vi "HOST.vi"() -> ()   [LabVIEW 2018]
uses:
  <vilib>/userdefined/High Color/nirio_resource_hc.ctl
  <instrlib>/niDCPower/nidcpower.llb/niDCPower Measurement Type.ctl
  <vilib>/FPGAPlugInAG/PXI-7953R/niLvFpga_Open_PXI-7953R.vi
  <vilib>/rvi/interface/common/dynamic/niFpgaDynamicAddResources.vi
  <vilib>/FPGAPlugInAG/Dynamic/niLvFpga_Reset_Dynamic.vi
  <vilib>/FPGAPlugInAG/Dynamic/niLvFpga_Run_Dynamic.vi
  <vilib>/Utility/error.llb/Error Cluster From Error Code.vi
  <vilib>/rvi/errors/niLvFpgaAdjustHostInterfaceError.vi
  <vilib>/FPGAPlugInAG/Dynamic/niLvFpga_Close_Dynamic.vi
  <vilib>/rvi/interface/nirviOpenFPGA/nirviOpenFPGA.xnode
  FPGA Bitfiles/MT9V024IA7XTM_FPGATarget_Target_SM0JNh2yPhg.lvbitx
  <vilib>/rvi/interface/nirviMethod/nirviMethod.xnode
  <vilib>/rvi/interface/nirviReadWriteControl/nirviReadWriteControl.xnode
  <vilib>/rvi/interface/nirviCloseFPGA/nirviCloseFPGA.xnode
  <vilib>/rvi/interface/Simulation/niFpgaSimulationCallBeginRW.vi
  <vilib>/FPGAPlugInAG/Dynamic/niLvFpga_ReadFifo_Dynamic.vi
  <vilib>/rvi/errors/niLvFpgaMergeErrorWithErrorCode.vi
  NiFpgaLv.dll
  <vilib>/Analysis/NI_AALBase.lvlib
panel:
  in  "Tab Control":enum32{"Основной", "Служебный"}(tab)
  out "Номер образца":string="0"
  in  "SEL 2":path=path "C:/LabView_PRJ/MT9V024IA7XTM/SEL"
  in  "resource name":T1="PXI1Slot6"
  in  "VAA_PIX":refnum<k15>="PXI1Slot3" caption="instrument handle"
  in  "VDD_LVDS":refnum<k15>="PXI1Slot2" caption="instrument handle"
  in  "Стоп":bool
  in  "Питание":bool
  out "VDD Chart":dbl(graph)=-7.930775234089577 caption="Waveform Chart 5"
  out "VAA Chart":dbl(graph)=0.06968054713639742
  out "LVDS Chart":dbl(graph)=0.00048817553524479985
  out "VAA_cur, A":dbl caption="measurement" format="%_6g"
  in  "VAA_curlim, A":dbl=0.1 caption="current limit" format="%_6p"
  in  "VAA, V":dbl=3.3 caption="voltage level" format="%_6p"
  in  "LVDS, V":dbl=3.3 caption="voltage level" format="%_6p"
  out "LVDS_cur, A":dbl caption="measurement" format="%_6g"
  out "VDD_cur, A":dbl caption="measurement" format="%_6g"
  in  "LVDS_curlim, A":dbl=0.1 caption="current limit" format="%_6p"
  in  "VDD_curlim, A":dbl=0.1 caption="current limit" format="%_6p"
  in  "VDD, V":dbl=3.3 caption="voltage level" format="%_6p"
  out "PIX Chart":dbl(graph)=-0.009814653457617957
  out "PIX_cur, A":dbl caption="measurement" format="%_6g"
  in  "PIX_curlim, A":dbl=0.1 caption="current limit" format="%_6p"
  in  "PIX, V":dbl=3.3 caption="voltage level" format="%_6p"
  in  "ON/OFF":bool
  in  "STANDBY":bool
  in  "nRESET_BAR":bool
  in  "VDD_selcur":dbl=0.075 caption="current limit" format="%_6p"
  in  "LVDS_selcur":dbl=0.075 caption="current limit" format="%_6p"
  in  "VAA_selcur":dbl=0.075 caption="current limit" format="%_6p"
  in  "PIX_selcur":dbl=0.075 caption="current limit" format="%_6p"
  out "VDD 2":bool
  out "LVDS 2":bool
  out "VAA 2":bool
  out "PIX 2":bool
  out "VDD":u32
  out "LVDS":u32
  out "VAA":u32
  out "PIX":u32
  in  "Период, мс":u32=100
  in  "SIM_SEL":bool
  out "SEL":bool
  out "REG_WR":bool
  in  "Получить кадр":bool
  in  "Непрерывно":bool=TRUE
  in  "SEL_T, мс":u32=100
  in  "Прошивка":bool
  in  "SAVE":bool
  in  "ПРИМЕЧАНИЕ":string
  in  "Светлый (T)\nТемный (F)":bool
  in  "Запись(T)/Чтение(F)":bool
  out "Image":T2(plugin-control)
  out "READ":u16=16 format="%x"
  in  "Регистр":u8=7 format="%x"
  in  "Данные":u16=920 format="%x"
  in  "Запись":u16=184 format="%x"
  out "Записали адресов":u32=360960
  out "世男":bool
  in  "Frames":path=path "C:/LabView_PRJ/MT9V024IA7XTM/FRAMES"
  out "СКО, ед.":u16=13
  out "СЗ, ед":u16=891
  in  "Со стороны":bool
  in  "Анализ":path=path "C:/Users/agest/Downloads/MT9V024IA7XTM/MT9V024IA7XTM/FRAMES/Первый кадр.PNG"
  in  "Write":bool[](array[boolean])=[FALSE, FALSE, FALSE, FALSE, FALSE, FALSE, FALSE, FALSE, TRUE, FALSE, FALSE, TRUE, TRUE, TRUE, FALSE, TRUE, FALSE, FALSE, TRUE, FALSE, FALSE, TRUE, FALSE, FALSE, FALSE, FALSE, FALSE, FALSE, FALSE, FALSE, TRUE, TRUE, TRUE, FALSE, TRUE]
  out "Array":bool[](array[boolean])=[TRUE, TRUE, TRUE, TRUE, TRUE, TRUE, TRUE, TRUE, FALSE, FALSE, FALSE, FALSE, FALSE, FALSE, FALSE, FALSE, FALSE, FALSE, TRUE, TRUE, FALSE, TRUE, FALSE, FALSE, FALSE, FALSE, FALSE, FALSE, FALSE, FALSE, TRUE, TRUE, TRUE, FALSE, TRUE, FALSE, FALSE, FALSE, FALSE, FALSE, FALSE, FALSE, FALSE]
  out "Read":bool[](array[boolean])=[FALSE, FALSE, FALSE, FALSE, TRUE, FALSE, FALSE, FALSE, TRUE, FALSE, FALSE, FALSE, FALSE, FALSE, FALSE, FALSE, FALSE]
  out "array w/ subset deleted":bool[](array[boolean])=[FALSE, FALSE, FALSE, FALSE, TRUE, FALSE, FALSE, FALSE, FALSE, FALSE, FALSE, FALSE, FALSE, FALSE, FALSE, FALSE]
  in  "Адресмассив":u8[](array[numeric])=[7, 175, 32, 112, 13, 15] format="%x"
  in  "Данныемассив":u16[](array[numeric])=[920, 0, 453, 1, 784, 257] format="%x"
  out "Data":u16[][](array[numeric])
  # "7 - 398\nAF - 0\n20 - 1C5\n70 - 1\nD - 310\nB - 10 (1 мс)\nB - 627 (100 мс)"
  # "D0"
  # "D7"
  # "\"0\""
  # "D8"
  # "D15"
  # "\"0\""
  # "R0"
  # "R7"
  # "\"0\""
  # "А0"
  # "\"В8\" - запись"
  # "А7"
  # "А0"
  # "St"
  # "\"0\""
  # "R0"
  # "R7"
  # "\"0\""
  # "А0"
  # "\"В8\" - запись"
  # "А7"
  # "А7"
  # "\"В9\" - чтение"
  # "0"
  # "35"
  # "Режим \"Запись\""
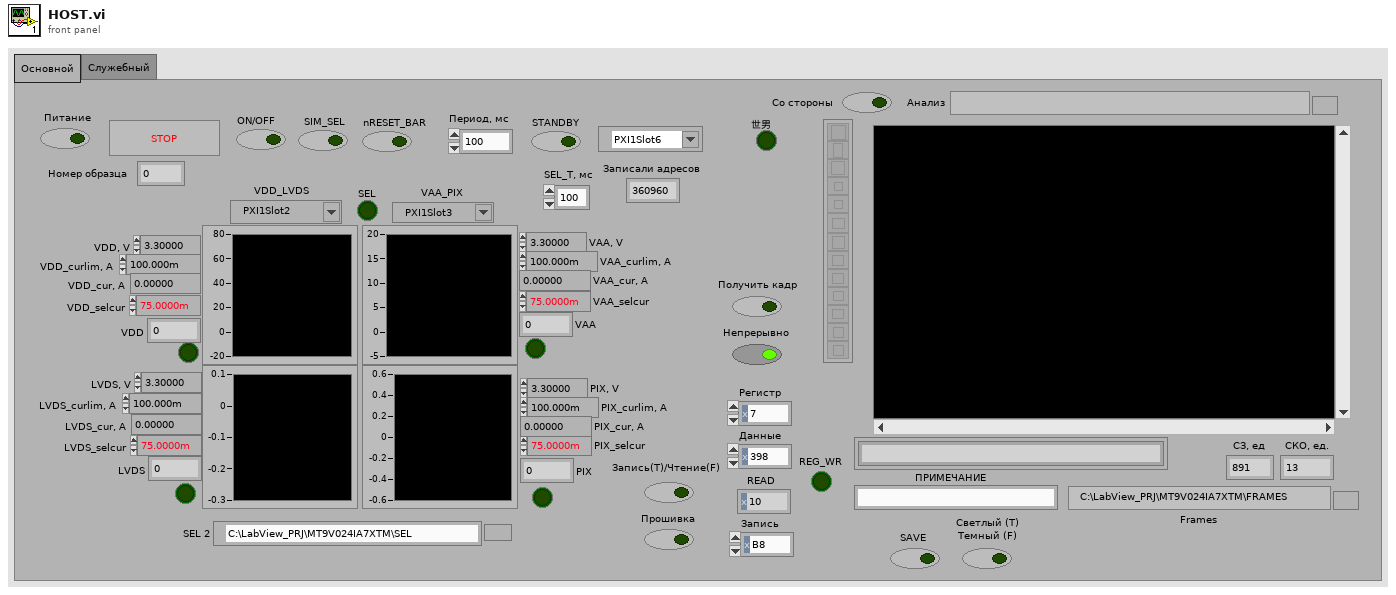
[diagram p1: front panel]
types:
  T1 = typedef "nirio_resource_hc.ctl" = tag
  T2 = typedef "IMAQ Image.ctl" = refnum<image>
  T3 = typedef "Image Type" = u32
  T4 = enum16{"open", "replace", "create", "open or create", "replace or create", "replace or create with confirmation"}
  T5 = typedef "niDCPower Measurement Type.ctl" = i32
  T6 = cluster{"Global Rectangle":i32[], "Contours":cluster{"Contour Type":u32, "ROI Type":u32, "Points":i32[]}[]}
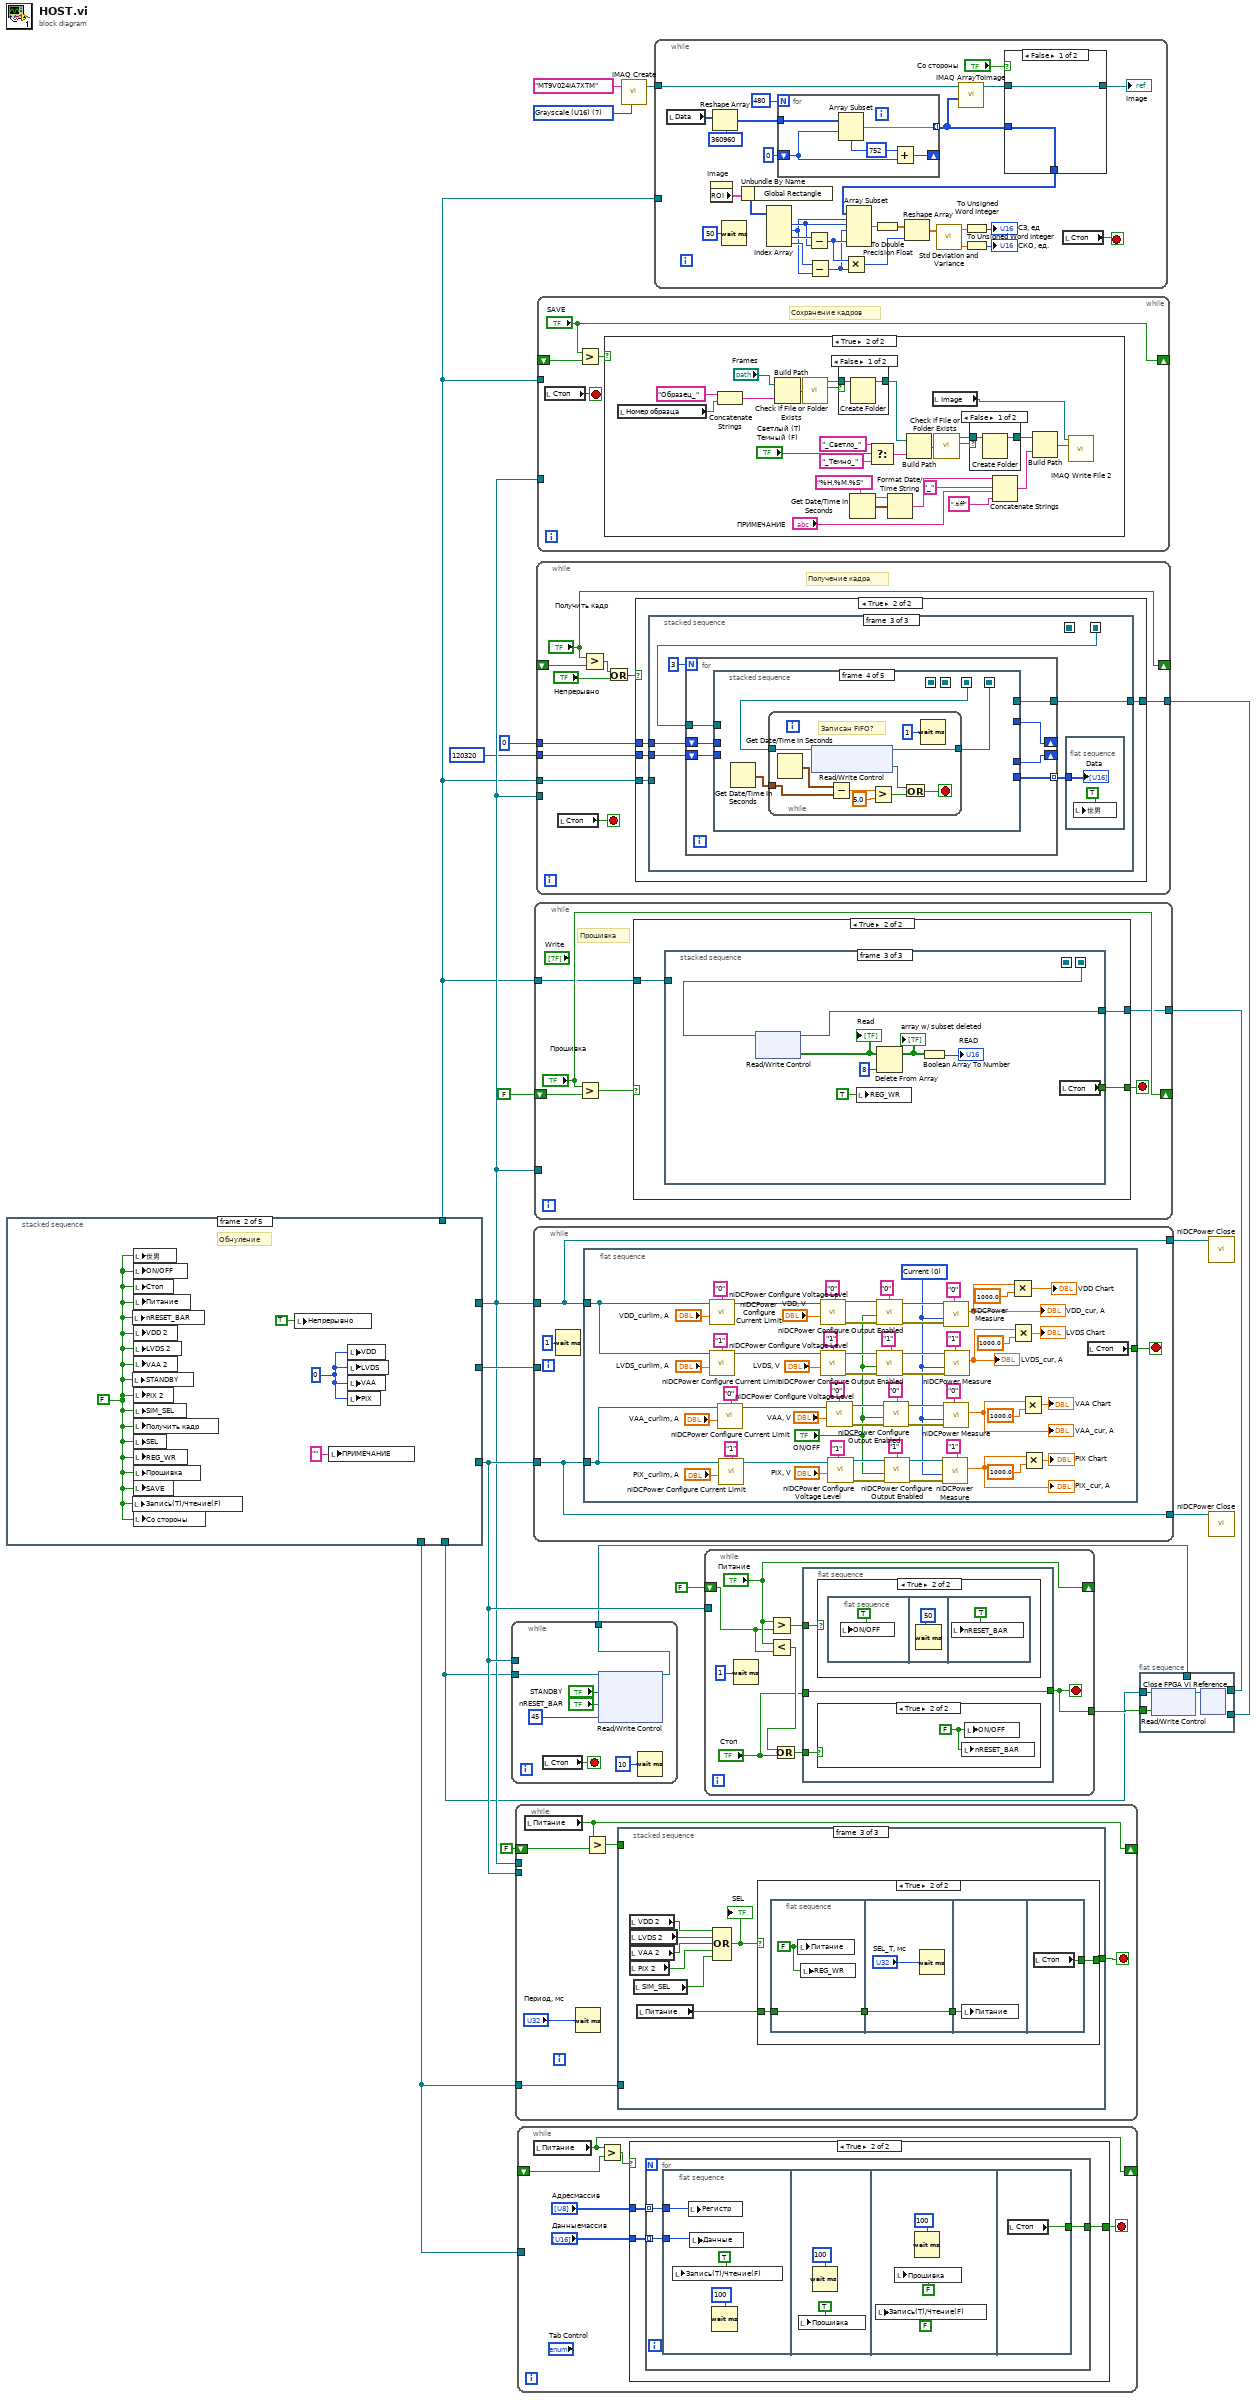
[diagram p0: block diagram]
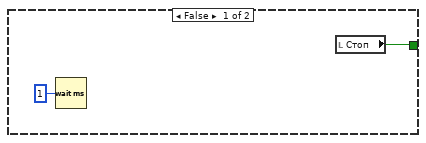
[diagram p2: hidden frame]
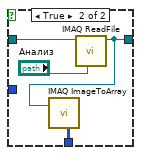
[diagram p3: hidden frame]
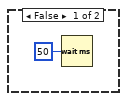
[diagram p4: hidden frame]
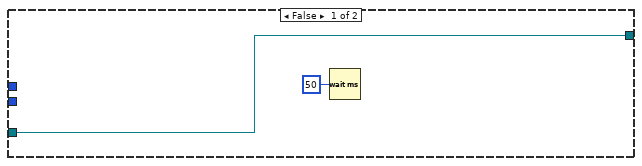
[diagram p7: hidden frame]
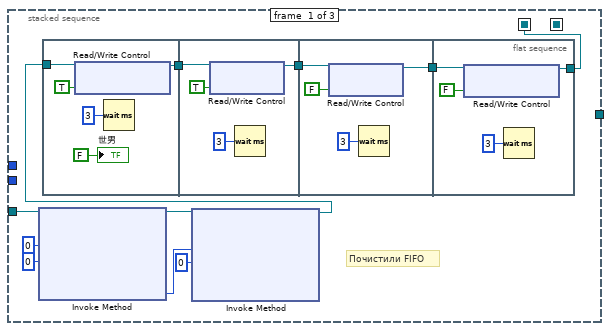
[diagram p8: hidden frame]
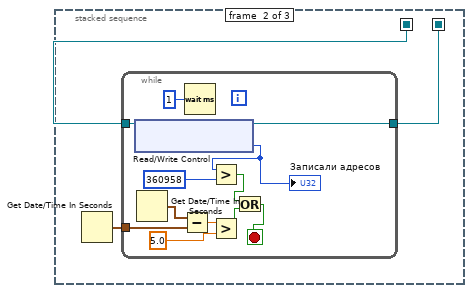
[diagram p9: hidden frame]
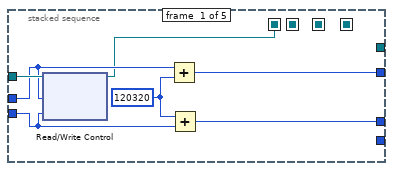
[diagram p10: hidden frame]
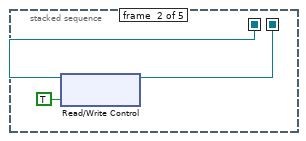
[diagram p11: hidden frame]
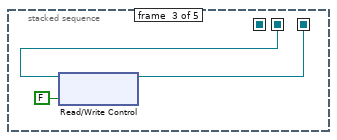
[diagram p12: hidden frame]
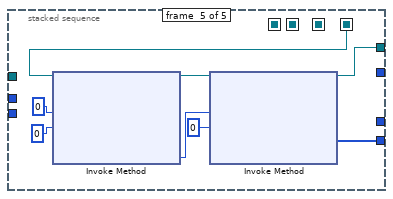
[diagram p13: hidden frame]
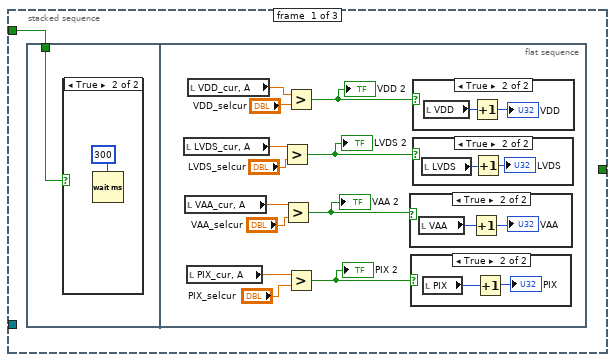
[diagram p14: hidden frame]
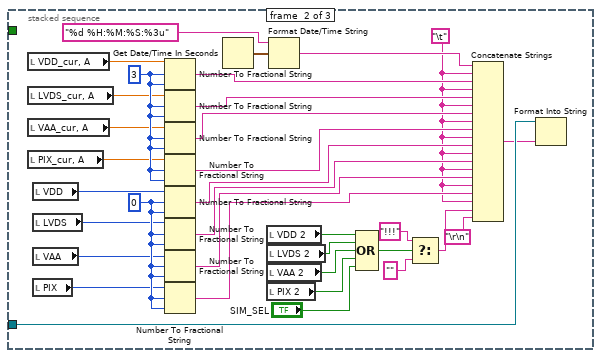
[diagram p20: hidden frame]
diagram:
  w8 = T3 7 items=["Grayscale (U8)", "Grayscale (I16)", "Grayscale (SGL)", "Complex (CSG)", "RGB (U32)", "HSL (U32)", "RGB (U64)", "Grayscale (U16)"] ("Image Type")
  n1 = stacked-sequence {
    tunnel: [_ _ w26 _ _] -> w3
    tunnel: [_ _ _ w62 _] -> w13
    tunnel: [_ _ _ _ w69] -> w12
    tunnel: [_ _ _ _ w68] -> w16
    tunnel: [_ _ _ w62 _] -> w4
    tunnel: [_ _ _ w62 _] -> w2
    frame #0 {
      # "Begin"
      n2 = call "Begin.vi"() -> ("Номер образца 2"=→"Номер образца":string)  [unwired: 11 in]
    }
    frame #1 {
      w25 = u32 0
      w22 = FALSE
      # "Обнуление"
      n3 = local write "nRESET_BAR"(w22) -> ()
      n4 = local write "STANDBY"(w22) -> ()
      n5 = local write "Запись(T)/Чтение(F)"(w22) -> ()
      n6 = local write "世男"(w22) -> ()
      n7 = local write "ON/OFF"(w22) -> ()
      n8 = local write "Стоп"(w22) -> ()
      n9 = local write "Питание"(w22) -> ()
      n10 = local write "VDD 2"(w22) -> ()
      n11 = local write "LVDS 2"(w22) -> ()
      n12 = local write "VAA 2"(w22) -> ()
      n13 = local write "PIX 2"(w22) -> ()
      n14 = local write "SIM_SEL"(w22) -> ()
      n15 = local write "Получить кадр"(w22) -> ()
      n16 = local write "SEL"(w22) -> ()
      n17 = local write "REG_WR"(w22) -> ()
      n18 = local write "Прошивка"(w22) -> ()
      n19 = local write "SAVE"(w22) -> ()
      n20 = local write "Со стороны"(w22) -> ()
      n21 = local write "Непрерывно"(TRUE ("Непрерывно")) -> ()
      n22 = local write "ПРИМЕЧАНИЕ"("" ("ПРИМЕЧАНИЕ")) -> ()
      n23 = local write "VDD"(w25) -> ()
      n24 = local write "LVDS"(w25) -> ()
      n25 = local write "VAA"(w25) -> ()
      n26 = local write "PIX"(w25) -> ()
    }
    frame #2 {
      w29 = "\t"
      # "Инициализаци первой строки лога по токам"
      n27 = local read "Номер образца"() -> (w35:string)
      n28 = Build Path(base path="SEL 2", name or relative path=w35) -> (appended path=w33:path)
      n29 = Get Date/Time In Seconds() -> (seconds since 1Jan1904=w40:timestamp)
      n30 = call <vilib>:"Check if File or Folder Exists.vi"("path"=w33) -> ("file or folder exists?"=w32:bool, "dup path"=w31:path)  [unwired: 8 in, 1 out]
      n31 = Format Date/Time String(time format string (%c)="%d %H.%M.%S", seconds (now)=w40) -> (date/time string=w43:string)  [unwired: 1 in]
      n32 = case shown="False" w32 {
        tunnel: w31 -> [w60 w61]
        tunnel: [w59 w61] -> w47
        frame False {
          n33 = Create Folder(path (use dialog)=w60) -> (created path=w59:path)  [unwired: 2 in, 2 out]
        }
        frame True {
        }
      }
      n34 = Concatenate Strings(w43, ".xls" ("string")) -> (w45:string)
      n35 = Build Path(base path=w47, name or relative path=w45) -> (appended path=w42:path)
      n36 = Open/Create/Replace File(file path (use dialog)=w42, operation (0:open)=T4."open or create", access (0:read/write)=enum16{"read/write", "read-only", "write-only"}."read/write") -> (refnum out=w39:refnum<file>)  [unwired: 3 in, 2 out]
      n37 = case shown="True" TRUE {
        tunnel: w39 -> [w55 w58]
        tunnel: [w55 w56] -> w46
        frame False {
        }
        frame True {
          n38 = Set File Position(refnum=w58, from (0:start)=enum16{"start", "end", "current"}."end") -> (refnum out=w56:refnum<file>)  [unwired: 2 in, 1 out]
        }
      }
      n39 = Format Into String(initial string=w46, "Time" ("input 1"), w29, "VDD_cur" ("input 1"), w29, "VDDLVDS_cur" ("input 1"), w29, "VAA_cur" ("input 1"), w29, "VAAPIX_cur" ("input 1"), w29, "VDD_sel" ("input 1"), w29, "VDDLVDS_sel" ("input 1"), w29, "VAA_sel" ("input 1"), w29, "VAAPIX_sel" ("input 1"), "\r\n") -> (resulting string=w26:refnum<file>)  [unwired: 2 in, 1 out]
    }
    frame #3 {
      n40 = xnode "Open FPGA VI Reference"("resource name"="resource name") -> ("FPGA VI Reference Out"=w63:refnum<k20>, "error out"=w65:errorcluster)  [unwired: 1 in]
      n41 = xnode "Invoke Method"("FPGA VI Reference In"=w63, "error in"=w65) -> ("FPGA VI Reference Out"=w66:refnum<k20>, "error out"=w64:errorcluster)
      n42 = xnode "Invoke Method"("FPGA VI Reference In"=w66, "error in"=w64) -> ("FPGA VI Reference Out"=w62:refnum<k20>)  [unwired: 1 in, 1 out]
    }
    frame #4 {
      n43 = call <instrlib>:"niDCPower Initialize.vi"("resource name"="VDD_LVDS") -> ("error out"=w73:errorcluster, "instrument handle out"=w71:refnum<k15>)  [unwired: 3 in, 6 out]
      n44 = call <instrlib>:"niDCPower Initialize.vi"("resource name"="VAA_PIX") -> ("error out"=w72:errorcluster, "instrument handle out"=w70:refnum<k15>)  [unwired: 3 in, 6 out]
      n45 = call <instrlib>:"niDCPower Configure Voltage Level.vi"("error in (no error)"=w73, "voltage level"=0.0, "channel name"="0,1", "instrument handle"=w71) -> ("instrument handle out"=w69:refnum<k15>)  [unwired: 6 in, 1 out]
      n46 = call <instrlib>:"niDCPower Configure Voltage Level.vi"("error in (no error)"=w72, "voltage level"=0.0, "channel name"="0,1", "instrument handle"=w70) -> ("instrument handle out"=w68:refnum<k15>)  [unwired: 6 in, 1 out]
    }
  }
  n47 = while {
    tunnel: w4 -> [w85]
    tunnel: w16 -> [_]
    tunnel: [w80] -> w7
    stop <- w86 stop-if-true
    n48 = local read "Стоп"() -> (w86:bool)
    n49 = xnode "Read/Write Control"("FPGA VI Reference In"=w85, "STANDBY"="STANDBY", "RESET_BAR"="nRESET_BAR", "46"=u8 45) -> ("FPGA VI Reference Out"=w80:refnum<k20>)  [unwired: 1 in, 1 out]
    n50 = Wait (ms)(milliseconds to wait=u32 10) -> ()  [unwired: 1 out]
  }
  n51 = while {
    tunnel: w16 -> [_]
    tunnel: w12 -> [_]
    shift-right: [w91] -> _
    shift-left: FALSE ("Питание") -> [w92]
    tunnel: w3 -> [w87]
    stop <- w89 stop-if-true
    n52 = local read "Питание"() -> (w91:bool)
    n53 = Wait (ms)(milliseconds to wait="Период, мс") -> ()  [unwired: 1 out]
    n54 = Greater?(x=w91, y=w92) -> (0:w90:bool)
    n55 = stacked-sequence {
      tunnel: w90 -> [w93 _ _]
      tunnel: [_ _ w151] -> w89
      tunnel: w87 -> [_ w146 _]
      frame #0 {
        n56 = flat-sequence {
          tunnel: w93 -> [w94]
          frame #0 {
            n57 = case shown="True" w94 {
              frame False {
              }
              frame True {
                n58 = Wait (ms)(milliseconds to wait=u32 300) -> ()  [unwired: 1 out]
              }
            }
          }
          frame #1 {
            n59 = local read "LVDS_cur, A"() -> (w105:dbl)
            n60 = local read "VAA_cur, A"() -> (w103:dbl)
            n61 = local read "PIX_cur, A"() -> (w101:dbl)
            n62 = local read "VDD_cur, A"() -> (w107:dbl)
            n63 = Greater?(x=w105, y="LVDS_selcur") -> (0:w96:bool)
            "LVDS 2" <- w96
            n64 = Greater?(x=w103, y="VAA_selcur") -> (0:w98:bool)
            "VAA 2" <- w98
            n65 = Greater?(x=w107, y="VDD_selcur") -> (0:w97:bool)
            "VDD 2" <- w97
            n66 = Greater?(x=w101, y="PIX_selcur") -> (0:w99:bool)
            "PIX 2" <- w99
            n67 = case shown="True" w98 {
              frame False {
              }
              frame True {
                n68 = local read "VAA"() -> (w113:u32)
                n69 = Increment(x=w113) -> (x+1=→"VAA":u32)
              }
            }
            n70 = case shown="True" w99 {
              frame False {
              }
              frame True {
                n71 = local read "PIX"() -> (w111:u32)
                n72 = Increment(x=w111) -> (x+1=→"PIX":u32)
              }
            }
            n73 = case shown="True" w97 {
              frame False {
              }
              frame True {
                n74 = local read "VDD"() -> (w115:u32)
                n75 = Increment(x=w115) -> (x+1=→"VDD":u32)
              }
            }
            n76 = case shown="True" w96 {
              frame False {
              }
              frame True {
                n77 = local read "LVDS"() -> (w109:u32)
                n78 = Increment(x=w109) -> (x+1=→"LVDS":u32)
              }
            }
          }
        }
      }
      frame #1 {
        w148 = i16 0 ("width (-)")
        w147 = i16 3 ("width (-)")
        w123 = "\t"
        n79 = local read "VDD_cur, A"() -> (w144:dbl)
        n80 = local read "LVDS_cur, A"() -> (w143:dbl)
        n81 = local read "VAA_cur, A"() -> (w142:dbl)
        n82 = local read "PIX_cur, A"() -> (w141:dbl)
        n83 = local read "VDD"() -> (w119:u32)
        n84 = local read "LVDS"() -> (w118:u32)
        n85 = local read "VAA"() -> (w117:u32)
        n86 = local read "PIX"() -> (w116:u32)
        n87 = Number To Fractional String(number=w144, width (-)=w147, precision (6)=w147) -> (F-format string=w131:string)  [unwired: 1 in]
        n88 = Number To Fractional String(number=w143, width (-)=w147, precision (6)=w147) -> (F-format string=w130:string)  [unwired: 1 in]
        n89 = Number To Fractional String(number=w142, width (-)=w147, precision (6)=w147) -> (F-format string=w129:string)  [unwired: 1 in]
        n90 = Number To Fractional String(number=w141, width (-)=w147, precision (6)=w147) -> (F-format string=w128:string)  [unwired: 1 in]
        n91 = Number To Fractional String(number=w119, width (-)=w148, precision (6)=w148) -> (F-format string=w127:string)  [unwired: 1 in]
        n92 = Number To Fractional String(number=w118, width (-)=w148, precision (6)=w148) -> (F-format string=w126:string)  [unwired: 1 in]
        n93 = Number To Fractional String(number=w117, width (-)=w148, precision (6)=w148) -> (F-format string=w125:string)  [unwired: 1 in]
        n94 = Number To Fractional String(number=w116, width (-)=w148, precision (6)=w148) -> (F-format string=w124:string)  [unwired: 1 in]
        n95 = Get Date/Time In Seconds() -> (seconds since 1Jan1904=w145:timestamp)
        n96 = local read "VDD 2"() -> (w140:bool)
        n97 = local read "LVDS 2"() -> (w139:bool)
        n98 = local read "VAA 2"() -> (w138:bool)
        n99 = local read "PIX 2"() -> (w137:bool)
        n100 = Format Date/Time String(time format string (%c)="%d %H:%M:%S:%3u", seconds (now)=w145) -> (date/time string=w132:string)  [unwired: 1 in]
        n101 = Compound Arithmetic op=OR(w140, w139, w138, w137, "SIM_SEL") -> (w133:bool)
        n102 = Select(t="!!!", s=w133, f="") -> (s? t:f=w122:string)
        n103 = Concatenate Strings(w132, w123, w131, w123, w130, w123, w129, w123, w128, w123, w127, w123, w126, w123, w125, w123, w124, w123, w122, "\r\n") -> (w120:string)
        n104 = Format Into String(initial string=w146, w120) -> ()  [unwired: 2 in, 2 out]
      }
      frame #2 {
        n105 = local read "VDD 2"() -> (w157:bool)
        n106 = local read "LVDS 2"() -> (w156:bool)
        n107 = local read "VAA 2"() -> (w155:bool)
        n108 = local read "PIX 2"() -> (w154:bool)
        n109 = local read "SIM_SEL"() -> (w153:bool)
        n110 = local read "Питание"() -> (w150:bool)
        n111 = Compound Arithmetic op=OR(w157, w156, w155, w154, w153) -> (w152:bool)
        "SEL" <- w152
        n112 = case shown="True" w152 {
          tunnel: [w158 w162] -> w151
          tunnel: w150 -> [_ w159]
          frame False {
            n113 = local read "Стоп"() -> (w158:bool)
          }
          frame True {
            n114 = flat-sequence {
              tunnel: [w163] -> w160
              tunnel: w159 -> [w163]
              tunnel: [w165] -> w161
              tunnel: w160 -> [w165]
              tunnel: w161 -> [w167]
              tunnel: [w168] -> w162
              frame #0 {
                w164 = FALSE ("Питание")
                n115 = local write "Питание"(w164) -> ()
                n116 = local write "REG_WR"(w164) -> ()
              }
              frame #1 {
                n117 = Wait (ms)(milliseconds to wait="SEL_T, мс") -> ()  [unwired: 1 out]
              }
              frame #2 {
                n118 = local write "Питание"(w167) -> ()
              }
              frame #3 {
                n119 = local read "Стоп"() -> (w168:bool)
              }
            }
          }
        }
      }
    }
  }
  n120 = while {
    tunnel: w3 -> [_]
    shift-right: [w172] -> _
    shift-left: _ -> [w174]
    stop <- w171 stop-if-true
    n121 = local read "Питание"() -> (w172:bool)
    n122 = Greater?(x=w172, y=w174) -> (0:w173:bool)
    n123 = case shown="True" w173 {
      tunnel: [w175 w179] -> w171
      tunnel: "Адресмассив" -> [_ w178]
      tunnel: "Данныемассив" -> [_ w177]
      frame False {
        n124 = Wait (ms)(milliseconds to wait=u32 1) -> ()  [unwired: 1 out]
        n125 = local read "Стоп"() -> (w175:bool)
      }
      frame True {
        n126 = for {
          tunnel: [w182] -> w179
          tunnel: w178 -> [w181] mode=indexing
          tunnel: w177 -> [w180] mode=indexing
          n127 = flat-sequence {
            tunnel: w181 -> [w184]
            tunnel: w180 -> [w183]
            tunnel: [w192] -> w182
            frame #0 {
              n128 = local write "Запись(T)/Чтение(F)"(TRUE ("Запись(T)/Чтение(F)")) -> ()
              n129 = local write "Регистр"(w184) -> ()
              n130 = local write "Данные"(w183) -> ()
              n131 = Wait (ms)(milliseconds to wait=u32 100) -> ()  [unwired: 1 out]
            }
            frame #1 {
              n132 = local write "Прошивка"(TRUE ("Прошивка")) -> ()
              n133 = Wait (ms)(milliseconds to wait=u32 100) -> ()  [unwired: 1 out]
            }
            frame #2 {
              n134 = local write "Запись(T)/Чтение(F)"(FALSE ("Запись(T)/Чтение(F)")) -> ()
              n135 = local write "Прошивка"(FALSE ("Прошивка")) -> ()
              n136 = Wait (ms)(milliseconds to wait=u32 100) -> ()  [unwired: 1 out]
            }
            frame #3 {
              n137 = local read "Стоп"() -> (w192:bool)
            }
          }
        }
      }
    }
  }
  n138 = while {
    tunnel: w16 -> [w193]
    tunnel: w12 -> [w194]
    tunnel: [w194] -> w18
    tunnel: [w193] -> w19
    tunnel: w13 -> [_]
    stop <- w195 stop-if-true
    n139 = Wait (ms)(milliseconds to wait=u32 1) -> ()  [unwired: 1 out]
    n140 = flat-sequence {
      tunnel: w194 -> [w216]
      tunnel: w193 -> [w202]
      tunnel: [w214] -> w195
      frame #0 {
        w201 = T5 0 items=["Current", "Voltage"] ("measurement type")
        n141 = call <instrlib>:"niDCPower Configure Current Limit.vi"("current limit"="VDD_curlim, A", "channel name"="0", "instrument handle"=w216) -> ("instrument handle out"=w247:refnum<k15>)  [unwired: 7 in, 1 out]
        n142 = call <instrlib>:"niDCPower Configure Current Limit.vi"("current limit"="LVDS_curlim, A", "channel name"="1", "instrument handle"=w216) -> ("instrument handle out"=w248:refnum<k15>)  [unwired: 7 in, 1 out]
        n143 = call <instrlib>:"niDCPower Configure Current Limit.vi"("current limit"="VAA_curlim, A", "channel name"="0", "instrument handle"=w202) -> ("instrument handle out"=w230:refnum<k15>)  [unwired: 7 in, 1 out]
        n144 = call <instrlib>:"niDCPower Configure Current Limit.vi"("current limit"="PIX_curlim, A", "channel name"="1", "instrument handle"=w202) -> ("instrument handle out"=w207:refnum<k15>)  [unwired: 7 in, 1 out]
        n145 = call <instrlib>:"niDCPower Configure Voltage Level.vi"("voltage level"="VDD, V", "channel name"="0", "instrument handle"=w247) -> ("error out"=w240:errorcluster, "instrument handle out"=w243:refnum<k15>)  [unwired: 7 in]
        n146 = call <instrlib>:"niDCPower Configure Voltage Level.vi"("voltage level"="LVDS, V", "channel name"="1", "instrument handle"=w248) -> ("error out"=w241:errorcluster, "instrument handle out"=w242:refnum<k15>)  [unwired: 7 in]
        n147 = call <instrlib>:"niDCPower Configure Voltage Level.vi"("voltage level"="VAA, V", "channel name"="0", "instrument handle"=w230) -> ("error out"=w234:errorcluster, "instrument handle out"=w235:refnum<k15>)  [unwired: 7 in]
        n148 = call <instrlib>:"niDCPower Configure Voltage Level.vi"("voltage level"="PIX, V", "channel name"="1", "instrument handle"=w207) -> ("error out"=w205:errorcluster, "instrument handle out"=w204:refnum<k15>)  [unwired: 7 in]
        n149 = call <instrlib>:"niDCPower Configure Output Enabled.vi"("error in (no error)"=w240, "output enabled"="ON/OFF", "channel name"="0", "instrument handle"=w243) -> ("error out"=w252:errorcluster, "instrument handle out"=w251:refnum<k15>)  [unwired: 6 in]
        n150 = call <instrlib>:"niDCPower Configure Output Enabled.vi"("error in (no error)"=w241, "output enabled"="ON/OFF", "channel name"="1", "instrument handle"=w242) -> ("error out"=w253:errorcluster, "instrument handle out"=w254:refnum<k15>)  [unwired: 6 in]
        n151 = call <instrlib>:"niDCPower Configure Output Enabled.vi"("error in (no error)"=w234, "output enabled"="ON/OFF", "channel name"="0", "instrument handle"=w235) -> ("error out"=w226:errorcluster, "instrument handle out"=w227:refnum<k15>)  [unwired: 6 in]
        n152 = call <instrlib>:"niDCPower Configure Output Enabled.vi"("error in (no error)"=w205, "output enabled"="ON/OFF", "channel name"="1", "instrument handle"=w204) -> ("error out"=w210:errorcluster, "instrument handle out"=w209:refnum<k15>)  [unwired: 6 in]
        n153 = call <instrlib>:"niDCPower Measure.vi"("error in (no error)"=w210, "measurement type"=w201, "channel name"="1", "instrument handle"=w209) -> ("measurement"=w213:dbl)  [unwired: 5 in, 2 out]
        "PIX_cur, A" <- w213
        n154 = call <instrlib>:"niDCPower Measure.vi"("error in (no error)"=w252, "measurement type"=w201, "channel name"="0", "instrument handle"=w251) -> ("measurement"=w219:dbl)  [unwired: 5 in, 2 out]
        "VDD_cur, A" <- w219
        n155 = call <instrlib>:"niDCPower Measure.vi"("error in (no error)"=w226, "measurement type"=w201, "channel name"="0", "instrument handle"=w227) -> ("measurement"=w220:dbl)  [unwired: 5 in, 2 out]
        "VAA_cur, A" <- w220
        n156 = call <instrlib>:"niDCPower Measure.vi"("error in (no error)"=w253, "measurement type"=w201, "channel name"="1", "instrument handle"=w254) -> ("measurement"=w222:dbl)  [unwired: 5 in, 2 out]
        "LVDS_cur, A" <- w222
        n157 = Multiply(x=w219, y=1000.0) -> (x*y=→"VDD Chart":dbl)
        n158 = Multiply(x=w222, y=1000.0) -> (x*y=→"LVDS Chart":dbl)
        n159 = Multiply(x=w220, y=1000.0) -> (x*y=→"VAA Chart":dbl)
        n160 = Multiply(x=w213, y=1000.0) -> (x*y=→"PIX Chart":dbl)
        n161 = local read "Стоп"() -> (w214:bool)
      }
    }
  }
  n162 = while {
    shift-right: ["Прошивка"] -> _
    shift-left: FALSE ("Прошивка") -> [w263]
    tunnel: w12 -> [_]
    tunnel: w2 -> [w260]
    tunnel: [w259] -> w6
    stop <- w261 stop-if-true
    # "Прошивка"
    n163 = Greater?(x="Прошивка", y=w263) -> (0:w258:bool)
    n164 = case shown="True" w258 {
      tunnel: [w265 w269] -> w261
      tunnel: w260 -> [w264 w268]
      tunnel: [w264 w267] -> w259
      frame False {
        n165 = Wait (ms)(milliseconds to wait=u32 1) -> ()  [unwired: 1 out]
        n166 = local read "Стоп"() -> (w265:bool)
      }
      frame True {
        n167 = stacked-sequence {
          seq-local: [w270 _ _] -> [_ w302 _]
          seq-local: [_ w301 _] -> [_ _ w314]
          tunnel: [_ _ w319] -> w269
          tunnel: w268 -> [w288 _ _]
          tunnel: [_ _ w313] -> w267
          frame #0 {
            n168 = Increment(x="Запись") -> (x+1=w272:u16)
            n169 = Multiply(x=u16 256, y=w272) -> (x*y=w281:u16)
            n170 = Number To Boolean Array(number="Запись") -> (Boolean array=w282:bool[])
            n171 = Number To Boolean Array(number="Данные") -> (Boolean array=w279:bool[])
            n172 = Number To Boolean Array(number="Регистр") -> (Boolean array=w283:bool[])
            n173 = Number To Boolean Array(number=w281) -> (Boolean array=w284:bool[])
            n174 = Delete From Array(array=w279, length=8, index=8) -> (deleted portion=w275:bool[], array with subset deleted=w276:bool[])
            n175 = case shown="False" "Запись(T)/Чтение(F)" {
              tunnel: FALSE -> [w291 w297]
              tunnel: w284 -> [w290 _]
              tunnel: w283 -> [w293 w300]
              tunnel: w282 -> [w294 w298]
              tunnel: [w292 w299] -> w280
              tunnel: w276 -> [_ w296]
              tunnel: w275 -> [_ w295]
              frame False {
                n176 = Build Array (concatenate)(w290, w291, w291, w293, w291, w294) -> (w292:bool[])
              }
              frame True {
                n177 = Build Array (concatenate)(w296, w297, w295, w297, w300, w297, w298) -> (w299:bool[])
              }
            }
            "Array" <- w280
            n178 = xnode "Read/Write Control"("FPGA VI Reference In"=w288, "Write"=w280, "Запись(T)/Чтение(F)"="Запись(T)/Чтение(F)") -> ("FPGA VI Reference Out"=w270:refnum<k20>)  [unwired: 1 in, 1 out]
            "REG_WR" <- FALSE ("REG_WR")
          }
          frame #1 {
            # "Цикл записи всех интересующих нас регистров"
            n179 = flat-sequence {
              tunnel: [w306] -> w303
              tunnel: w302 -> [w305]
              tunnel: [w309] -> w304
              tunnel: w303 -> [w309]
              tunnel: w304 -> [w312]
              tunnel: [w310] -> w301
              frame #0 {
                n180 = xnode "Read/Write Control"("FPGA VI Reference In"=w305, "Регистр"=TRUE) -> ("FPGA VI Reference Out"=w306:refnum<k20>)  [unwired: 1 in, 1 out]
              }
              frame #1 {
                n181 = Wait (ms)(milliseconds to wait=u32 1) -> ()  [unwired: 1 out]
              }
              frame #2 {
                n182 = xnode "Read/Write Control"("FPGA VI Reference In"=w312, "Регистр"=FALSE) -> ("FPGA VI Reference Out"=w310:refnum<k20>)  [unwired: 1 in, 1 out]
              }
            }
          }
          frame #2 {
            n183 = xnode "Read/Write Control"("FPGA VI Reference In"=w314) -> ("FPGA VI Reference Out"=w313:refnum<k20>, "Read"=w316:bool[])  [unwired: 1 in, 1 out]
            "Read" <- w316
            n184 = local write "REG_WR"(TRUE ("REG_WR")) -> ()
            n185 = Delete From Array(array=w316, index=8) -> (array with subset deleted=w315:bool[])  [unwired: 1 in, 1 out]
            "array w/ subset deleted" <- w315
            n186 = Boolean Array To Number(Boolean array=w315) -> (number=→"READ":u16)
            n187 = local read "Стоп"() -> (w319:bool)
          }
        }
      }
    }
  }
  n188 = while {
    tunnel: w12 -> [_]
    tunnel: w2 -> [w324]
    shift-right: ["Получить кадр"] -> _
    shift-left: _ -> [w329]
    tunnel: u32 0 -> [w323]
    tunnel: u32 120320 ("163840") -> [w322]
    tunnel: [w321] -> w5
    stop <- w330 stop-if-true
    # "Получение кадра"
    n189 = local read "Стоп"() -> (w330:bool)
    n190 = Greater?(x="Получить кадр", y=w329) -> (0:w326:bool)
    n191 = Or(x=w326, y="Непрерывно") -> (x .or. y?=w325:bool)
    n192 = case shown="True" w325 {
      tunnel: w324 -> [w331 w336]
      tunnel: w323 -> [_ w335]
      tunnel: w322 -> [_ w334]
      tunnel: [w331 w333] -> w321
      frame False {
        n193 = Wait (ms)(milliseconds to wait=u32 50) -> ()  [unwired: 1 out]
      }
      frame True {
        n194 = stacked-sequence {
          seq-local: [w337 _ _] -> [_ w366 _]
          seq-local: [_ w365 _] -> [_ _ w381]
          tunnel: w336 -> [w343 _ _]
          tunnel: w335 -> [_ _ w384]
          tunnel: w334 -> [_ _ w383]
          tunnel: [_ _ w380] -> w333
          frame #0 {
            # "Почистили FIFO"
            n195 = xnode "Invoke Method"("FPGA VI Reference In"=w343, "Number of Elements"=u32 0, "Timeout (ms)"=0) -> ("FPGA VI Reference Out"=w342:refnum<k20>, "Elements Remaining"=w344:u32)  [unwired: 1 in, 2 out]
            n196 = flat-sequence {
              tunnel: w341 -> [w352]
              tunnel: [w349] -> w340
              tunnel: w340 -> [w355]
              tunnel: [w353] -> w339
              tunnel: w339 -> [w359]
              tunnel: [w358] -> w338
              tunnel: w338 -> [w363]
              tunnel: [w361] -> w337
              frame #0 {
                n197 = xnode "Read/Write Control"("FPGA VI Reference In"=w352, "Кадр в память"=TRUE ("EXPOSURE")) -> ("FPGA VI Reference Out"=w349:refnum<k20>)  [unwired: 1 in, 1 out]
                n198 = Wait (ms)(milliseconds to wait=u32 3) -> ()  [unwired: 1 out]
                "世男" <- FALSE
              }
              frame #1 {
                n199 = xnode "Read/Write Control"("FPGA VI Reference In"=w355, "EXPOSURE"=TRUE) -> ("FPGA VI Reference Out"=w353:refnum<k20>)  [unwired: 1 in, 1 out]
                n200 = Wait (ms)(milliseconds to wait=u32 3) -> ()  [unwired: 1 out]
              }
              frame #2 {
                n201 = xnode "Read/Write Control"("FPGA VI Reference In"=w359, "EXPOSURE"=FALSE) -> ("FPGA VI Reference Out"=w358:refnum<k20>)  [unwired: 1 in, 1 out]
                n202 = Wait (ms)(milliseconds to wait=u32 3) -> ()  [unwired: 1 out]
              }
              frame #3 {
                n203 = xnode "Read/Write Control"("FPGA VI Reference In"=w363, "Кадр в память"=FALSE) -> ("FPGA VI Reference Out"=w361:refnum<k20>)  [unwired: 1 in, 1 out]
                n204 = Wait (ms)(milliseconds to wait=u32 3) -> ()  [unwired: 1 out]
              }
            }
            n205 = xnode "Invoke Method"("FPGA VI Reference In"=w342, "Number of Elements"=w344, "Timeout (ms)"=0) -> ("FPGA VI Reference Out"=w341:refnum<k20>)  [unwired: 1 in, 3 out]
          }
          frame #1 {
            n206 = Get Date/Time In Seconds() -> (seconds since 1Jan1904=w367:timestamp)
            n207 = while {
              tunnel: [w378] -> w365
              tunnel: w366 -> [w377]
              tunnel: w367 -> [w374]
              stop <- w369 stop-if-true
              n208 = xnode "Read/Write Control"("FPGA VI Reference In"=w377) -> ("FPGA VI Reference Out"=w378:refnum<k20>, "Записали адресов"=w368:u32)  [unwired: 1 in, 1 out]
              "Записали адресов" <- w368
              n209 = Get Date/Time In Seconds() -> (seconds since 1Jan1904=w375:timestamp)
              n210 = Subtract(x=w375, y=w374) -> (x-y=w373:dbl)
              n211 = Wait (ms)(milliseconds to wait=u32 1) -> ()  [unwired: 1 out]
              n212 = Greater?(x=w368, y=u32 360958) -> (0:w371:bool)
              n213 = Greater?(x=w373, y=5.0) -> (0:w370:bool)
              n214 = Or(x=w371, y=w370) -> (x .or. y?=w369:bool)
            }
          }
          frame #2 {
            n215 = for {
              N: 3 -> [_]
              tunnel: w381 -> [w394]
              shift-right: [w391] -> _
              shift-left: w384 -> [w393]
              shift-right: [w390] -> _
              shift-left: w383 -> [w392]
              tunnel: [w389] -> w382 mode=indexing
              tunnel: [w388] -> w380
              n216 = stacked-sequence {
                seq-local: [w395 _ _ _ _] -> [_ w403 _ _ _]
                seq-local: [_ w402 _ _ _] -> [_ _ w406 _ _]
                seq-local: [_ _ w405 _ _] -> [_ _ _ w410 _]
                seq-local: [_ _ _ w409 _] -> [_ _ _ _ w421]
                tunnel: w394 -> [w401 _ _ _ _]
                tunnel: w393 -> [w399 _ _ _ _]
                tunnel: w392 -> [w398 _ _ _ _]
                tunnel: [w397 _ _ _ _] -> w391
                tunnel: [w396 _ _ _ _] -> w390
                tunnel: [_ _ _ _ w423] -> w389
                tunnel: [_ _ _ _ w422] -> w388
                frame #0 {
                  w400 = u32 120320 ("163840")
                  n217 = xnode "Read/Write Control"("FPGA VI Reference In"=w401, "Нач_адр"=w399, "Кон_адр"=w398) -> ("FPGA VI Reference Out"=w395:refnum<k20>)  [unwired: 1 in, 1 out]
                  n218 = Add(x=w399, y=w400) -> (x+y=w397:u32)
                  n219 = Add(x=w400, y=w398) -> (x+y=w396:u32)
                }
                frame #1 {
                  n220 = xnode "Read/Write Control"("FPGA VI Reference In"=w403, "Кадр на ПК"=TRUE ("HOST")) -> ("FPGA VI Reference Out"=w402:refnum<k20>)  [unwired: 1 in, 1 out]
                }
                frame #2 {
                  n221 = xnode "Read/Write Control"("FPGA VI Reference In"=w406, "Кадр на ПК"=FALSE ("HOST")) -> ("FPGA VI Reference Out"=w405:refnum<k20>)  [unwired: 1 in, 1 out]
                }
                frame #3 {
                  n222 = Get Date/Time In Seconds() -> (seconds since 1Jan1904=w408:timestamp)
                  n223 = while {
                    tunnel: w410 -> [w419]
                    tunnel: [w418] -> w409
                    tunnel: w408 -> [w416]
                    stop <- w411 stop-if-true
                    # "Записан FIFO?"
                    n224 = Get Date/Time In Seconds() -> (seconds since 1Jan1904=w417:timestamp)
                    n225 = xnode "Read/Write Control"("FPGA VI Reference In"=w419) -> ("FPGA VI Reference Out"=w418:refnum<k20>, "Записали FIFO"=w413:bool)  [unwired: 1 in, 1 out]
                    n226 = Subtract(x=w417, y=w416) -> (x-y=w415:dbl)
                    n227 = Greater?(x=w415, y=5.0) -> (0:w412:bool)
                    n228 = Or(x=w413, y=w412) -> (x .or. y?=w411:bool)
                    n229 = Wait (ms)(milliseconds to wait=u32 1) -> ()  [unwired: 1 out]
                  }
                }
                frame #4 {
                  n230 = xnode "Invoke Method"("FPGA VI Reference In"=w421, "Number of Elements"=u32 0, "Timeout (ms)"=0) -> ("FPGA VI Reference Out"=w427:refnum<k20>, "Elements Remaining"=w428:u32)  [unwired: 1 in, 2 out]
                  n231 = xnode "Invoke Method"("FPGA VI Reference In"=w427, "Number of Elements"=w428, "Timeout (ms)"=0) -> ("FPGA VI Reference Out"=w422:refnum<k20>, "Data"=w423:u16[])  [unwired: 1 in, 2 out]
                }
              }
            }
            n232 = flat-sequence {
              tunnel: w382 -> [w387]
              frame #0 {
                n233 = local write "世男"(TRUE) -> ()
                "Data" <- w387
              }
            }
          }
        }
      }
    }
  }
  n234 = while {
    tunnel: w12 -> [_]
    tunnel: w2 -> [_]
    shift-right: ["SAVE"] -> _
    shift-left: _ -> [w431]
    stop <- w432 stop-if-true
    # "Сохранение кадров"
    n235 = local read "Стоп"() -> (w432:bool)
    n236 = Greater?(x="SAVE", y=w431) -> (0:w429:bool)
    n237 = case shown="True" w429 {
      frame False {
        n238 = Wait (ms)(milliseconds to wait=u32 50) -> ()  [unwired: 1 out]
      }
      frame True {
        n239 = local read "Номер образца"() -> (w453:string)
        n240 = Concatenate Strings("Образец_" ("string"), w453) -> (w458:string)
        n241 = Build Path(base path="Frames", name or relative path=w458) -> (appended path=w455:path)
        n242 = call <vilib>:"Check if File or Folder Exists.vi"("path"=w455) -> ("file or folder exists?"=w456:bool, "dup path"=w457:path)  [unwired: 8 in, 1 out]
        n243 = case shown="False" w456 {
          tunnel: w457 -> [w463 w464]
          tunnel: [w462 w464] -> w437
          frame False {
            n244 = Create Folder(path (use dialog)=w463) -> (created path=w462:path)  [unwired: 2 in, 2 out]
          }
          frame True {
          }
        }
        n245 = Get Date/Time In Seconds() -> (seconds since 1Jan1904=w447:timestamp)
        n246 = Select(t="_Светло_", s="Светлый (T)\nТемный (F)", f="_Темно_") -> (s? t:f=w446:string)
        n247 = Format Date/Time String(time format string (%c)="%H.%M.%S", seconds (now)=w447) -> (date/time string=w443:string)  [unwired: 1 in]
        n248 = Build Path(base path=w437, name or relative path=w446) -> (appended path=w451:path)
        n249 = local read "Image"() -> (w436:T2)
        n250 = call <vilib>:"Check if File or Folder Exists.vi"("path"=w451) -> ("file or folder exists?"=w450:bool, "dup path"=w449:path)  [unwired: 8 in, 1 out]
        n251 = case shown="False" w450 {
          tunnel: w449 -> [w460 w461]
          tunnel: [w459 w461] -> w445
          frame False {
            n252 = Create Folder(path (use dialog)=w460) -> (created path=w459:path)  [unwired: 2 in, 2 out]
          }
          frame True {
          }
        }
        n253 = Concatenate Strings(w443, "_", "ПРИМЕЧАНИЕ", ".tiff" ("element")) -> (w444:string)
        n254 = Build Path(base path=w445, name or relative path=w444) -> (appended path=w448:path)
        n255 = call-poly "IMAQ Write File 2"("File Path"=w448, "Image"=w436) -> ()  [unwired: 8 in, 2 out]
      }
    }
  }
  n256 = call "IMAQ Create"("Image Name"="MT9V024IA7XTM", "Image Type"=w8) -> ("New Image"=w1:T2)  [unwired: 3 in, 1 out]
  n257 = while {
    tunnel: w2 -> [_]
    tunnel: w1 -> [w471]
    stop <- w493 stop-if-true
    n258 = local read "Data"() -> (w491:u16[][])
    n259 = property on="Image" class="ImageControl"() -> ("ROI"=w472:T6)  [unwired: 2 in, 2 out]
    n260 = Reshape Array(w491, 360960 ("dimension size")) -> (w490:u16[])
    n261 = Wait (ms)(milliseconds to wait=u32 50) -> ()  [unwired: 1 out]
    n262 = Unbundle By Name(w472) -> ("Global Rectangle"=w480:i32[])
    n263 = Index Array(array=w480) -> (element #1=w478:i32, element #2=w475:i32, element #3=w479:i32, element #4=w476:i32)  [unwired: 4 in]
    n264 = for {
      N: 480 ("length 2") -> [_]
      tunnel: w490 -> [w504]
      shift-right: [w503] -> _
      shift-left: 0 ("index") -> [w502]
      tunnel: [w501] -> w465 mode=indexing
      w500 = 752 ("length")
      n265 = Array Subset(array=w504, index=w502, length=w500) -> (w501:u16[])
      n266 = Add(x=w500, y=w502) -> (x+y=w503:i32)
    }
    n267 = Subtract(x=w479, y=w478) -> (x-y=w477:i32)
    n268 = Subtract(x=w476, y=w475) -> (x-y=w474:i32)
    n269 = Multiply(x=w477, y=w474) -> (x*y=w487:i32)
    n270 = call "IMAQ ArrayToImage"("Image Pixels (U16)"=w465, "Image"=w471) -> ("Image Out"=w467:T2)  [unwired: 8 in, 1 out]
    n271 = case shown="False" "Со стороны" {
      tunnel: [w495 w497] -> w468
      tunnel: w467 -> [w495 w498]
      tunnel: [w494 w496] -> w466
      tunnel: w465 -> [w494 _]
      frame False {
      }
      frame True {
        n272 = call "IMAQ ReadFile"("File Path"="Анализ", "Image"=w498) -> ("Image Out"=w497:T2)  [unwired: 5 in, 4 out]
        n273 = call "IMAQ ImageToArray"("Image"=w497) -> ("Image Pixels (U16)"=w496:u16[][])  [unwired: 3 in, 4 out]
      }
    }
    "Image" <- w468
    n274 = Array Subset(array=w466, index (row)=w475, length (row)=w474, index (col)=w478, length (col)=w477) -> (w473:u16[][])
    n275 = To Double Precision Float(number=w473) -> (double precision float=w484:dbl[][])
    n276 = Reshape Array(w484, w487) -> (w483:dbl[])
    n277 = call <vilib>:"Std Deviation and Variance.vi"("X"=w483) -> ("mean"=w485:dbl, "standard deviation"=w482:dbl)  [unwired: 1 in, 1 out]
    n278 = To Unsigned Word Integer(number=w485) -> (unsigned 16bit integer=→"СЗ, ед":u16)
    n279 = To Unsigned Word Integer(number=w482) -> (unsigned 16bit integer=→"СКО, ед.":u16)
    n280 = local read "Стоп"() -> (w493:bool)
  }
  n281 = while {
    shift-right: ["Питание"] -> _
    shift-left: FALSE -> [w511]
    tunnel: w16 -> [_]
    tunnel: [w505] -> w17
    stop <- w505 stop-if-true
    n282 = Wait (ms)(milliseconds to wait=u32 1) -> ()  [unwired: 1 out]
    n283 = Greater?(x="Питание", y=w511) -> (0:w510:bool)
    n284 = Less?(x="Питание", y=w511) -> (x < y?=w507:bool)
    n285 = Or(x=w507, y="Стоп") -> (x .or. y?=w508:bool)
    n286 = flat-sequence {
      tunnel: w508 -> [w515]
      tunnel: w510 -> [w514]
      tunnel: [w513] -> w505
      tunnel: "Стоп" -> [w513]
      frame #0 {
        n287 = case shown="True" w515 {
          frame False {
          }
          frame True {
            w516 = FALSE ("VDD18_ON")
            n288 = local write "nRESET_BAR"(w516) -> ()
            n289 = local write "ON/OFF"(w516) -> ()
          }
        }
        n290 = case shown="True" w514 {
          frame False {
          }
          frame True {
            n291 = flat-sequence {
              frame #0 {
                n292 = local write "ON/OFF"(TRUE ("VDD18_ON")) -> ()
              }
              frame #1 {
                n293 = Wait (ms)(milliseconds to wait=u32 50) -> ()  [unwired: 1 out]
              }
              frame #2 {
                n294 = local write "nRESET_BAR"(TRUE ("Автомат")) -> ()
              }
            }
          }
        }
      }
    }
  }
  n295 = flat-sequence {
    tunnel: w17 -> [w522]
    tunnel: w4 -> [w520]
    tunnel: w7 -> [_]
    tunnel: w6 -> [_]
    tunnel: w5 -> [_]
    frame #0 {
      n296 = xnode "Read/Write Control"("FPGA VI Reference In"=w520, "Стоп"=w522) -> ("FPGA VI Reference Out"=w521:refnum<k20>)  [unwired: 1 in, 1 out]
      n297 = xnode "Close FPGA VI Reference"("FPGA VI Reference In"=w521) -> ()  [unwired: 1 in, 1 out]
    }
  }
  n298 = call <instrlib>:"niDCPower Close.vi"("instrument handle"=w18) -> ()  [unwired: 10 in, 1 out]
  n299 = call <instrlib>:"niDCPower Close.vi"("instrument handle"=w19) -> ()  [unwired: 10 in, 1 out]
